vi "Write DAT (1D).vi"(4 "Append (0=F)":i32, 6 "Comments":string, 8 "error in":errorcluster, 9 "Data":dbl[](array[numeric]), 10 "Headers":string[](array[string]), 11 "path":path) -> (0 "error out":errorcluster, 3 "new file path":path)   [LabVIEW 2016, in "LV-Data.DAT.lvclass"]
uses:
  LV-Data.DAT.lvclass
  <vilib>/Utility/file.llb/Write Delimited Spreadsheet (string).vi
panel:
  out "appended array":string[][](array[string])
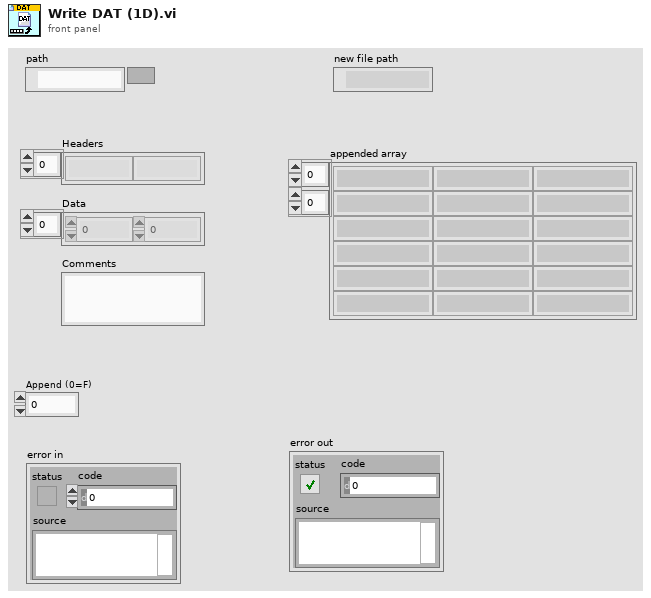
[diagram p1: front panel]
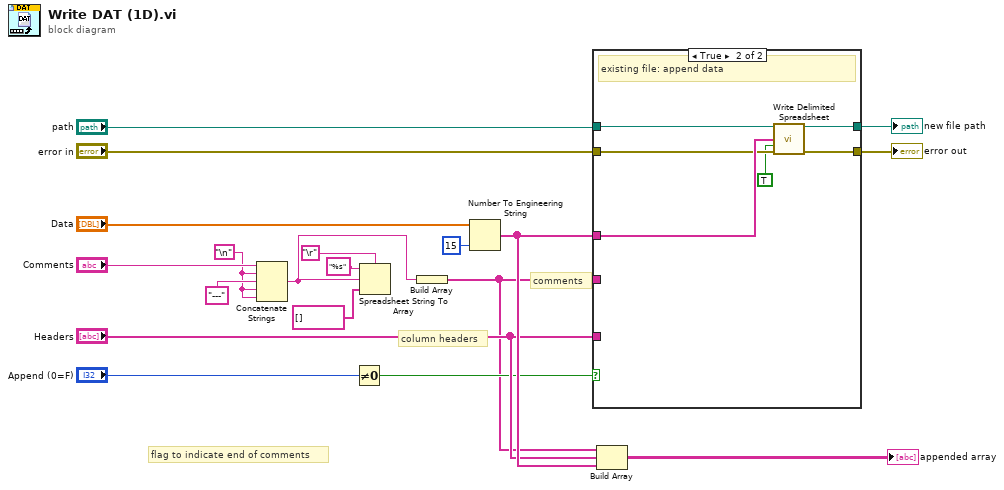
[diagram p0: block diagram]
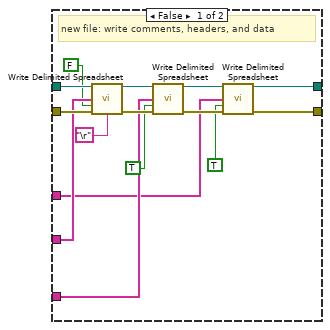
[diagram p2: hidden frame]
diagram:
  w8 = "\n"
  # "column headers"
  # "comments"
  # "flag to indicate end of comments"
  n1 = Concatenate Strings("Comments", w8, "---" ("string"), w8, w8) -> (w2:string)
  n2 = Not Equal To 0?(x="Append (0=F)") -> (x != 0?=w3:bool)
  n3 = Spreadsheet String To Array(delimiter (Tab)="\r", format string="%s", spreadsheet string=w2, array type (2D Dbl)=string[] []) -> ()  [unwired: 1 out]
  n4 = Build Array(w2) -> (w1:string[])
  n5 = Number To Engineering String(2:i16 15 ("precision (6)"), 4:"Data") -> (0:w6:string[])  [unwired: 2 out]
  n6 = case shown="True" w3 {
    tunnel: w1 -> [w29 _]
    tunnel: [w23 w37] -> w14
    tunnel: w6 -> [w21 w39]
    tunnel: "path" -> [w34 w40]
    tunnel: "error in" -> [w33 w38]
    tunnel: [w22 w36] -> w13
    tunnel: "Headers" -> [w24 _]
    frame False {
      # "new file: write comments, headers, and data"
      n7 = call-poly <vilib>:"Write Delimited Spreadsheet.vi"("file path (dialog if empty)"=w34, "1D data"=w29, "append to file? (new file:F)"=FALSE, "error in (no error)"=w33, "delimiter (\\t)"="\r") -> ("new file path (Not A Path if cancelled)"=w31:path, "error out"=w32:errorcluster)  [unwired: 9 in]
      n8 = call-poly <vilib>:"Write Delimited Spreadsheet.vi"("file path (dialog if empty)"=w31, "1D data"=w24, "append to file? (new file:F)"=TRUE, "error in (no error)"=w32) -> ("new file path (Not A Path if cancelled)"=w25:path, "error out"=w26:errorcluster)  [unwired: 10 in]
      n9 = call-poly <vilib>:"Write Delimited Spreadsheet.vi"("file path (dialog if empty)"=w25, "1D data"=w21, "append to file? (new file:F)"=TRUE, "error in (no error)"=w26) -> ("new file path (Not A Path if cancelled)"=w23:path, "error out"=w22:errorcluster)  [unwired: 10 in]
    }
    frame True {
      # "existing file: append data"
      n10 = call-poly <vilib>:"Write Delimited Spreadsheet.vi"("file path (dialog if empty)"=w40, "1D data"=w39, "append to file? (new file:F)"=TRUE, "error in (no error)"=w38) -> ("new file path (Not A Path if cancelled)"=w37:path, "error out"=w36:errorcluster)  [unwired: 10 in]
    }
  }
  "new file path" <- w14
  "error out" <- w13
  n11 = Build Array(w1, "Headers", w6) -> (→"appended array":string[][])
